vi "InsertOnMultipleWires.vi"(10 "Wire Array":refnum<vi>[](array[refnum]), 11 "To Insert":path) -> (2 "Inserted":refnum<vi>, 3 "Done?":bool)   [LabVIEW 2024, in "AddNewEvent.lvlib"]
uses:
  AddNewEvent.lvlib
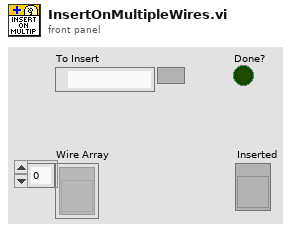
[diagram p1: front panel]
types:
  T1 = cluster{"Not Error Wire?":bool, "Source Term Top":i32, "Source Term Left":i32, "Wire Ref":refnum<vi>, "Source Term":refnum<vi>, "Sink Terms":refnum<vi>[], "Tried this one yet?":bool, "Sink Term Owner Owners":refnum<vi>[]}
  T2 = cluster{"Not Error Wire?":bool, "Source Term Top":i32, "Source Term Left":i32, "Wire Ref":refnum<vi>, "Source Term":refnum<vi>, "Sink Terms":refnum<vi>[], "Tried this one yet?":bool, "Sink Term Owner Owners":refnum<vi>[]}[]
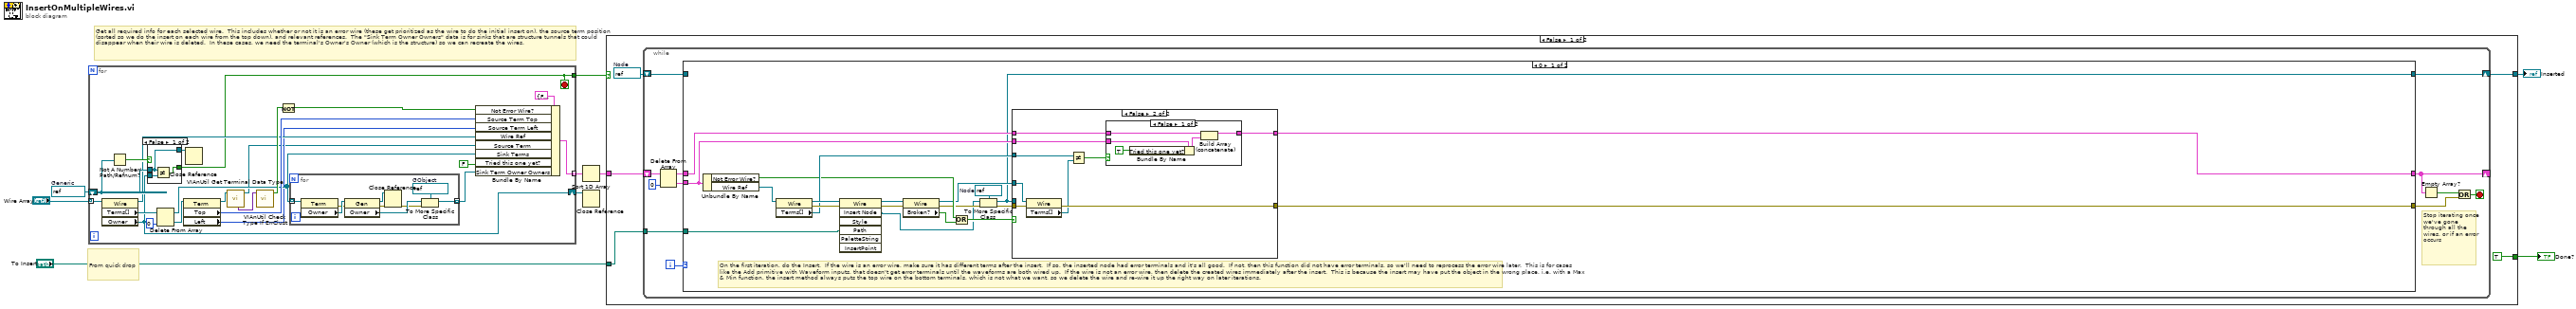
[diagram p0: block diagram]
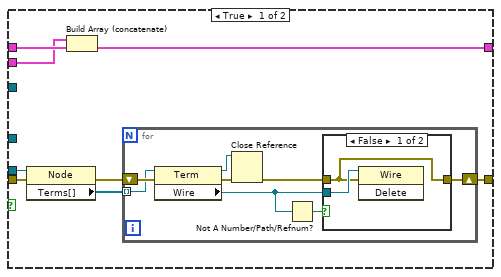
[diagram p2: hidden frame]
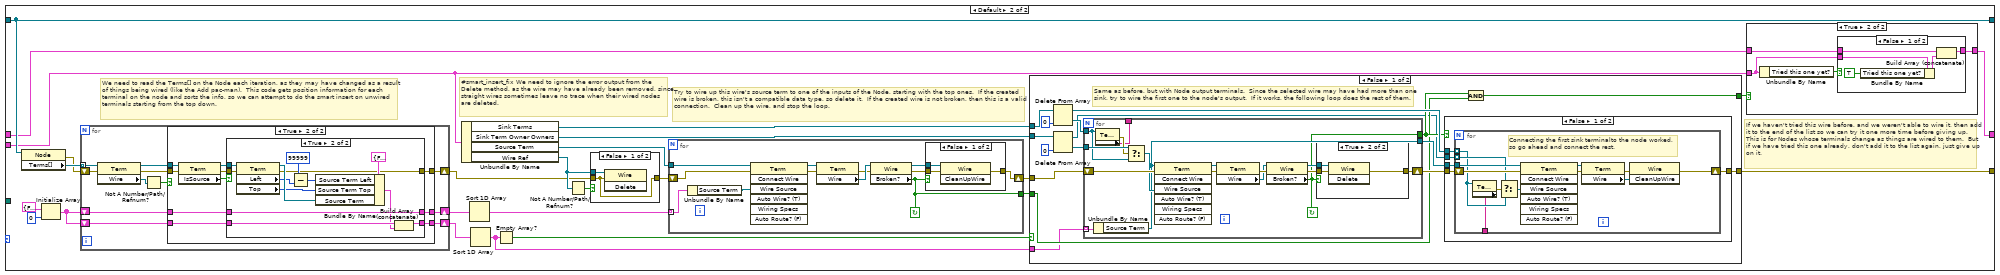
[diagram p5: hidden frame]
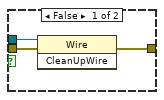
[diagram p8: hidden frame]
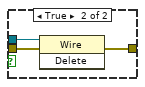
[diagram p12: hidden frame]
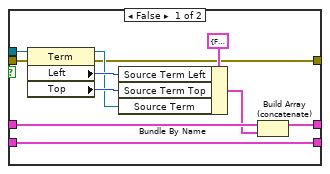
[diagram p14: hidden frame]
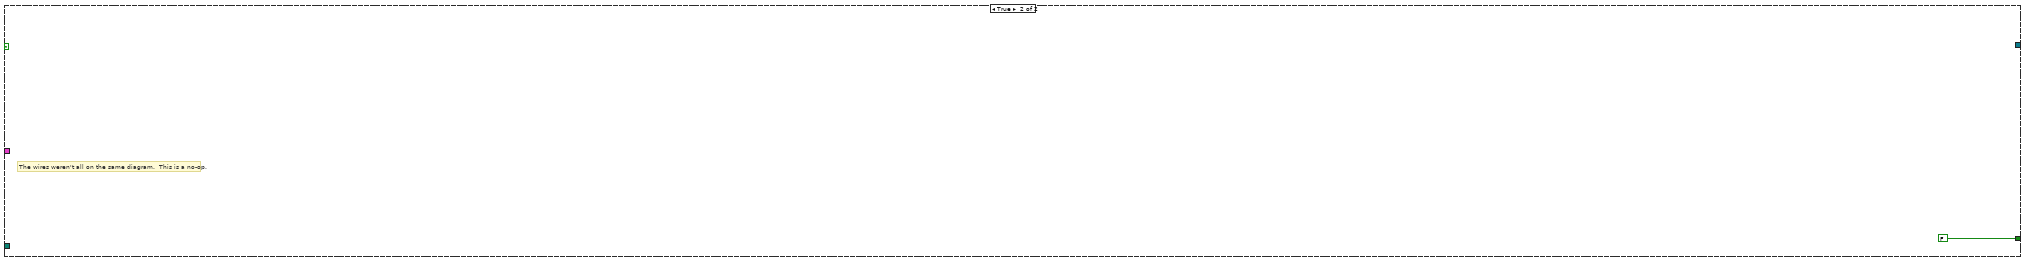
[diagram p15: hidden frame]
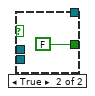
[diagram p16: hidden frame]
diagram:
  w6 = refnum<vi> refnum  # Generic
  # "From quick drop"
  # "Get all required info for each selected wire.  This includes whether or not it is an error wire (these get prioritized as the wire to do the initial insert on), the source term position (sorted so we do the insert on each wire from the top down), and relevant references.  The \"Sink Term Owner Owners\" data is for sinks that are structure tunnels that could disappear when their wire is deleted.  In these cases, we need the terminal's Owner's Owner (which is the structure) so we can recreate the wires."
  n1 = for {
    shift-right: [w16] -> w5
    shift-left: w6 -> [w31]
    tunnel: [w17] -> w7
    tunnel: "Wire Array" -> [w20] mode=indexing
    tunnel: [w19] -> w9 mode=indexing
    stop <- w17 stop-if-true
    n2 = property class="Wire"(reference=w20) -> (reference out=w23:refnum<vi>, "Terms[]"=w30:refnum<vi>[], "Owner"=w16:refnum<vi>)  [unwired: 1 in, 1 out]
    n3 = Not A Number/Path/Refnum?(number/path/refnum=w31) -> (NaN/Path/Refnum?=w28:bool)
    n4 = case shown="False" w28 {
      tunnel: [w42 FALSE] -> w17
      tunnel: w16 -> [w43 _]
      tunnel: w31 -> [w41 _]
      tunnel: [w41 _] -> w13
      frame False {
        n5 = Not Equal?(x=w41, y=w43) -> (x != y?=w42:bool)
      }
      frame True {
      }
    }
    n6 = Delete From Array(array=w30, index=0) -> (deleted portion=w18:refnum<vi>, array with subset deleted=w15:refnum<vi>[])  [unwired: 1 in]
    n7 = property class="Term"(reference=w18) -> (reference out=w12:refnum<vi>, "Top"=w25:i32, "Left"=w14:i32)  [unwired: 1 in, 1 out]
    n8 = Close Reference(reference=w13) -> ()  [unwired: 1 in, 1 out]
    n9 = call <vilib>:"VIAnUtil Get Terminal Data Type.vi"("Terminal in"=w12) -> ("Terminal out"=w11:refnum<vi>, "Type Variant"=w10:variant)  [unwired: 7 in, 2 out]
    n10 = call <vilib>:"VIAnUtil Check Type If ErrClust.vi"("Data In"=w10) -> ("IsErrClust?"=w26:bool)  [unwired: 1 in, 9 out]
    n11 = Not(x=w26) -> (.not. x?=w24:bool)
    n12 = for {
      tunnel: w15 -> [w40] mode=indexing
      tunnel: [w37] -> w21 mode=indexing
      w36 = refnum<vi> refnum  # GObject
      n13 = property class="Term"(reference=w40) -> (error out=w35:errorcluster, "Owner"=w39:refnum<vi>)  [unwired: 1 in, 1 out]
      n14 = property class="Gen"(reference=w39, error in=w35) -> (reference out=w33:refnum<vi>, error out=w34:errorcluster, "Owner"=w38:refnum<vi>)
      n15 = Close Reference(reference=w33, error in (no error)=w34) -> (error out=w32:errorcluster)
      n16 = To More Specific Class(target class=w36, reference=w38, error in=w32) -> (specific class reference=w37:refnum<vi>)  [unwired: 1 out]
    }
    n17 = Bundle By Name(cluster=T1 {"Not Error Wire?"=FALSE, "Source Term Top"=0, "Source Term Left"=0, "Wire Ref"=refnum, "Source Term"=refnum, "Sink Terms"=[], "Tried this one yet?"=FALSE, "Sink Term Owner Owners"=[]} ("Wire Information"), "Not Error Wire?"=w24, "Source Term Top"=w25, "Source Term Left"=w14, "Wire Ref"=w23, "Source Term"=w11, "Sink Terms"=w15, "Tried this one yet?"=FALSE, "Sink Term Owner Owners"=w21) -> (w19:T1)
  }
  n18 = Sort 1D Array(array=w9) -> (sorted array=w8:T2)
  n19 = Close Reference(reference=w5) -> ()  [unwired: 1 in, 1 out]
  n20 = case shown="False" w7 {
    tunnel: w8 -> [w49 _]
    tunnel: [TRUE FALSE] -> w2
    tunnel: "To Insert" -> [w46 _]
    tunnel: [w45 _] -> w1
    frame False {
      w48 = refnum<vi> refnum  # Node
      n21 = while {
        shift-right: [w59] -> _
        shift-left: w49 -> [w56]
        shift-right: [w51] -> w45
        shift-left: w48 -> [w58]
        tunnel: w46 -> [w52]
        i -> [w60]
        stop <- w53 stop-if-true
        # "Stop iterating once we've gone through all the wires, or if an error occurs"
        n22 = Delete From Array(array=w56, index=0) -> (deleted portion=w61:T1, array with subset deleted=w55:T2)  [unwired: 1 in]
        n23 = case shown="0" w60 {
          tunnel: w61 -> [w80 w125]
          tunnel: w55 -> [w68 w132]
          tunnel: [w62 w140] -> w51
          tunnel: [w81 w131] -> w59
          tunnel: w58 -> [_ w140]
          tunnel: [w79 w135] -> w50
          tunnel: w52 -> [w67 _]
          frame 0 {
            w65 = refnum<vi> refnum  # Node
            # "On the first iteration, do the Insert.  If the wire is an error wire, make sure it has different terms after the insert.  If so, the inserted node had error terminals and it's all good.  If not, then this function did not have error terminals, so we'll need to reprocess the error wire later.  This is for cases like the Add primitive with Waveform inputs, that doesn't get error terminals until the waveforms are both wired up.  If the wire is not an error wire, then delete the created wires immediately after the insert.  This is because the insert may have put the object in the wrong place, i.e. with a Max & Min function, the insert method always puts the top wire on the bottom terminals, which is not what we want, so we delete the wire and re-wire it up the right way on later iterations."
            n24 = Unbundle By Name(w80) -> ("Not Error Wire?"=w74:bool, "Wire Ref"=w78:refnum<vi>)
            n25 = property class="Wire"(reference=w78) -> (reference out=w76:refnum<vi>, error out=w77:errorcluster, "Terms[]"=w75:refnum<vi>[])  [unwired: 1 in]
            n26 = invoke class="Wire" method="Insert Node"(reference=w76, error in=w77, "Path"=w67) -> (reference out=w73:refnum<vi>, error out=w72:errorcluster, "Insert Node"=w63:refnum<vi>)  [unwired: 4 in, 4 out]
            n27 = property class="Wire"(reference=w73, error in=w72) -> (reference out=w71:refnum<vi>, error out=w66:errorcluster, "Broken?"=w70:bool)
            n28 = Or(x=w74, y=w70) -> (x .or. y?=w69:bool)
            n29 = To More Specific Class(target class=w65, reference=w63, error in=w66) -> (specific class reference=w62:refnum<vi>, error out=w64:errorcluster)
            n30 = case shown="False" w69 {
              tunnel: w68 -> [w89 w109]
              tunnel: [w87 w108] -> w81
              tunnel: w80 -> [w88 w107]
              tunnel: [w82 w104] -> w79
              tunnel: w64 -> [w84 w106]
              tunnel: w71 -> [_ w105]
              tunnel: w75 -> [_ w102]
              tunnel: w62 -> [w85 _]
              frame True {
                n31 = property class="Node"(reference=w85, error in=w84) -> (error out=w86:errorcluster, "Terms[]"=w83:refnum<vi>[])  [unwired: 1 out]
                n32 = Build Array (concatenate)(w88, w89) -> (w87:T2)
                n33 = for {
                  shift-right: [w91] -> w82
                  shift-left: w86 -> [w97]
                  tunnel: w83 -> [w96] mode=indexing
                  n34 = property class="Term"(reference=w96, error in=w97) -> (reference out=w94:refnum<vi>, error out=w95:errorcluster, "Wire"=w90:refnum<vi>)
                  n35 = Close Reference(reference=w94, error in (no error)=w95) -> (error out=w92:errorcluster)
                  n36 = Not A Number/Path/Refnum?(number/path/refnum=w90) -> (NaN/Path/Refnum?=w93:bool)
                  n37 = case shown="False" w93 {
                    tunnel: w92 -> [w98 w100]
                    tunnel: [w98 w100] -> w91
                    tunnel: w90 -> [w99 _]
                    frame False {
                      n38 = invoke class="Wire" method="Delete"(reference=w99, error in=w98) -> ()  [unwired: 1 in, 3 out]
                    }
                    frame True {
                    }
                  }
                }
              }
              frame False {
                n39 = property class="Wire"(reference=w105, error in=w106) -> (error out=w104:errorcluster, "Terms[]"=w103:refnum<vi>[])  [unwired: 1 out]
                n40 = Not Equal?(x=w102, y=w103) -> (x != y?=w101:bool)
                n41 = case shown="False" w101 {
                  tunnel: w109 -> [w114 w115]
                  tunnel: [w113 w115] -> w108
                  tunnel: w107 -> [w112 _]
                  frame False {
                    n42 = Bundle By Name(cluster=w112, "Tried this one yet?"=TRUE) -> (w111:T1)
                    n43 = Build Array (concatenate)(w114, w111) -> (w113:T2)
                  }
                  frame True {
                  }
                }
              }
            }
          }
          frame Default {
            # "#smart_insert_fix We need to ignore the error output from the Delete method, as the wire may have already been removed, since straight wires sometimes leave no trace when their wired nodes are deleted."
            # "If we haven't tried this wire before, and we weren't able to wire it, then add it to the end of the list so we can try it one more time before giving up.  This is for Nodes whose terminals change as things are wired to them.  But if we have tried this one already, don't add it to the list again, just give up on it."
            # "Try to wire up this wire's source term to one of the inputs of the Node, starting with the top ones.  If the created wire is broken, this isn't a compatible data type, so delete it.  If the created wire is not broken, then this is a valid connection.  Clean up the wire, and stop the loop."
            # "We need to read the Terms[] on the Node each iteration, as they may have changed as a result of things being wired (like the Add pac-man).  This code gets position information for each terminal on the node and sorts the info, so we can attempt to do the smart insert on unwired terminals starting from the top down."
            n44 = property class="Node"(reference=w140) -> (error out=w118:errorcluster, "Terms[]"=w139:refnum<vi>[])  [unwired: 1 in, 1 out]
            n45 = Initialize Array(T1 {"Not Error Wire?"=FALSE, "Source Term Top"=0, "Source Term Left"=0, "Wire Ref"=refnum, "Source Term"=refnum, "Sink Terms"=[], "Tried this one yet?"=FALSE, "Sink Term Owner Owners"=[]} ("Wire Information"), 0) -> (w119:T2)
            n46 = for {
              tunnel: w139 -> [w241] mode=indexing
              shift-right: [w237] -> w137
              shift-left: w119 -> [w240]
              shift-right: [w236] -> w136
              shift-left: w119 -> [w238]
              shift-right: [w231] -> w117
              shift-left: w118 -> [w233]
              n47 = property class="Term"(reference=w241, error in=w233) -> (reference out=w234:refnum<vi>, error out=w232:errorcluster, "Wire"=w235:refnum<vi>)
              n48 = Not A Number/Path/Refnum?(number/path/refnum=w235) -> (NaN/Path/Refnum?=w239:bool)
              n49 = case shown="True" w239 {
                tunnel: w240 -> [w244 w252]
                tunnel: w238 -> [w243 w251]
                tunnel: [w244 w249] -> w237
                tunnel: [w243 w250] -> w236
                tunnel: w234 -> [_ w254]
                tunnel: w232 -> [w242 w247]
                tunnel: [w242 w245] -> w231
                frame False {
                }
                frame True {
                  n50 = property class="Term"(reference=w254, error in=w247) -> (reference out=w248:refnum<vi>, error out=w246:errorcluster, "IsSource"=w253:bool)
                  n51 = case shown="True" w253 {
                    tunnel: w252 -> [w264 w276]
                    tunnel: w251 -> [w265 w278]
                    tunnel: [w265 w277] -> w250
                    tunnel: [w263 w276] -> w249
                    tunnel: w248 -> [w260 w275]
                    tunnel: w246 -> [w256 w268]
                    tunnel: [w255 w267] -> w245
                    frame False {
                      n52 = property class="Term"(reference=w260, error in=w256) -> (reference out=w257:refnum<vi>, error out=w255:errorcluster, "Left"=w259:i32, "Top"=w258:i32)
                      n53 = Bundle By Name(cluster=T1 {"Not Error Wire?"=FALSE, "Source Term Top"=0, "Source Term Left"=0, "Wire Ref"=refnum, "Source Term"=refnum, "Sink Terms"=[], "Tried this one yet?"=FALSE, "Sink Term Owner Owners"=[]} ("Wire Information"), "Source Term Left"=w259, "Source Term Top"=w258, "Source Term"=w257) -> (w261:T1)
                      n54 = Build Array (concatenate)(w264, w261) -> (w263:T2)
                    }
                    frame True {
                      n55 = property class="Term"(reference=w275, error in=w268) -> (reference out=w272:refnum<vi>, error out=w267:errorcluster, "Left"=w266:i32, "Top"=w271:i32)
                      n56 = Subtract(x=99999, y=w266) -> (x-y=w269:i32)
                      n57 = Bundle By Name(cluster=T1 {"Not Error Wire?"=FALSE, "Source Term Top"=0, "Source Term Left"=0, "Wire Ref"=refnum, "Source Term"=refnum, "Sink Terms"=[], "Tried this one yet?"=FALSE, "Sink Term Owner Owners"=[]} ("Wire Information"), "Source Term Left"=w269, "Source Term Top"=w271, "Source Term"=w272) -> (w273:T1)
                      n58 = Build Array (concatenate)(w278, w273) -> (w277:T2)
                    }
                  }
                }
              }
            }
            n59 = Unbundle By Name(w125) -> ("Sink Terms"=w124:refnum<vi>[], "Sink Term Owner Owners"=w123:refnum<vi>[], "Source Term"=w121:refnum<vi>, "Wire Ref"=w120:refnum<vi>)
            n60 = Sort 1D Array(array=w137) -> (sorted array=w130:T2)
            n61 = Sort 1D Array(array=w136) -> (sorted array=w129:T2)
            n62 = Empty Array?(array=w129) -> (empty?=w122:bool)
            n63 = Not A Number/Path/Refnum?(number/path/refnum=w120) -> (NaN/Path/Refnum?=w128:bool)
            n64 = case shown="False" w128 {
              tunnel: [w141 w143] -> w138
              tunnel: w120 -> [w142 _]
              tunnel: w117 -> [w141 w143]
              frame False {
                n65 = invoke class="Wire" method="Delete"(reference=w142, error in=w141) -> ()  [unwired: 1 in, 3 out]
              }
              frame True {
              }
            }
            n66 = for {
              tunnel: w121 -> [w224]
              tunnel: w130 -> [w223] mode=indexing
              tunnel: [w219] -> w133
              shift-right: [w213] -> w116
              shift-left: w138 -> [w217]
              stop <- w219 continue-if-true
              n67 = Unbundle By Name(w223) -> ("Source Term"=w218:refnum<vi>)
              n68 = invoke class="Term" method="Connect Wire"(reference=w224, error in=w217, "Wire Source"=w218) -> (reference out=w222:refnum<vi>, error out=w216:errorcluster)  [unwired: 4 in, 5 out]
              n69 = property class="Term"(reference=w222, error in=w216) -> (error out=w215:errorcluster, "Wire"=w221:refnum<vi>)  [unwired: 1 out]
              n70 = property class="Wire"(reference=w221, error in=w215) -> (reference out=w220:refnum<vi>, error out=w214:errorcluster, "Broken?"=w219:bool)
              n71 = case shown="False" w219 {
                tunnel: w220 -> [w227 w230]
                tunnel: w214 -> [w226 w229]
                tunnel: [w225 w228] -> w213
                frame False {
                  n72 = invoke class="Wire" method="CleanUpWire"(reference=w227, error in=w226) -> (error out=w225:errorcluster)  [unwired: 1 in, 2 out]
                }
                frame True {
                  n73 = invoke class="Wire" method="Delete"(reference=w230, error in=w229) -> (error out=w228:errorcluster)  [unwired: 1 in, 2 out]
                }
              }
            }
            n74 = case shown="False" w122 {
              tunnel: w124 -> [w159 _]
              tunnel: [w153 w200] -> w135
              tunnel: [w152 w201] -> w134
              tunnel: w133 -> [w150 w201]
              tunnel: w123 -> [w148 _]
              tunnel: w129 -> [w145 _]
              tunnel: w116 -> [w144 w200]
              frame False {
                # "Same as before, but with Node output terminals.  Since the selected wire may have had more than one sink, try to wire the first one to the node's output.  If it works, the following loop does the rest of them."
                n75 = Delete From Array(array=w159, index=0) -> (deleted portion=w157:refnum<vi>, array with subset deleted=w154:refnum<vi>[])  [unwired: 1 in]
                n76 = Delete From Array(array=w148, index=0) -> (deleted portion=w147:refnum<vi>, array with subset deleted=w146:refnum<vi>[])  [unwired: 1 in]
                n77 = for {
                  tunnel: w157 -> [w179]
                  tunnel: w145 -> [w184] mode=indexing
                  shift-right: [w186] -> w156
                  shift-left: w144 -> [w193]
                  tunnel: [w181] -> w151
                  tunnel: [w182] -> w155
                  tunnel: w147 -> [w185]
                  tunnel: [w178] -> _
                  stop <- w181 continue-if-true
                  n78 = Unbundle By Name(w184) -> ("Source Term"=w182:refnum<vi>)
                  n79 = property class="Term"(reference=w179) -> (error out=w180:errorcluster, "ClassName"=w178:string)  [unwired: 1 in, 1 out]
                  n80 = Select(t=w185, s=w180, f=w179) -> (s? t:f=w183:refnum<vi>)
                  n81 = invoke class="Term" method="Connect Wire"(reference=w182, error in=w193, "Wire Source"=w183) -> (reference out=w191:refnum<vi>, error out=w192:errorcluster)  [unwired: 4 in, 5 out]
                  n82 = property class="Term"(reference=w191, error in=w192) -> (error out=w190:errorcluster, "Wire"=w189:refnum<vi>)  [unwired: 1 out]
                  n83 = property class="Wire"(reference=w189, error in=w190) -> (reference out=w187:refnum<vi>, error out=w188:errorcluster, "Broken?"=w181:bool)
                  n84 = case shown="True" w181 {
                    tunnel: w188 -> [w196 w198]
                    tunnel: w187 -> [w195 w199]
                    tunnel: [w194 w197] -> w186
                    frame False {
                      n85 = invoke class="Wire" method="CleanUpWire"(reference=w195, error in=w196) -> (error out=w194:errorcluster)  [unwired: 1 in, 2 out]
                    }
                    frame True {
                      n86 = invoke class="Wire" method="Delete"(reference=w199, error in=w198) -> (error out=w197:errorcluster)  [unwired: 1 in, 2 out]
                    }
                  }
                }
                n87 = case shown="False" w151 {
                  tunnel: w156 -> [w164 w177]
                  tunnel: [w161 w177] -> w153
                  tunnel: w155 -> [w163 _]
                  tunnel: w154 -> [w162 _]
                  tunnel: w146 -> [w160 _]
                  frame False {
                    n88 = for {
                      tunnel: w163 -> [w175]
                      tunnel: w162 -> [w167] mode=indexing
                      shift-right: [w165] -> w161
                      shift-left: w164 -> [w176]
                      tunnel: w160 -> [w170] mode=indexing
                      tunnel: [w166] -> _
                      # "Connecting the first sink terminalto the node worked, so go ahead and connect the rest."
                      n89 = property class="Term"(reference=w167) -> (error out=w168:errorcluster, "ClassName"=w166:string)  [unwired: 1 in, 1 out]
                      n90 = Select(t=w170, s=w168, f=w167) -> (s? t:f=w169:refnum<vi>)
                      n91 = invoke class="Term" method="Connect Wire"(reference=w175, error in=w176, "Wire Source"=w169) -> (reference out=w174:refnum<vi>, error out=w173:errorcluster)  [unwired: 4 in, 5 out]
                      n92 = property class="Term"(reference=w174, error in=w173) -> (error out=w172:errorcluster, "Wire"=w171:refnum<vi>)  [unwired: 1 out]
                      n93 = invoke class="Wire" method="CleanUpWire"(reference=w171, error in=w172) -> (error out=w165:errorcluster)  [unwired: 1 in, 2 out]
                    }
                  }
                  frame True {
                    # "None of the node outputs would connect to this wire.  No need to try to process the rest of the sinks."
                  }
                }
                n94 = And(x=w151, y=w150) -> (x .and. y?=w152:bool)
              }
              frame True {
                # "There are no more unwired outputs on the node.  Don't bother trying to find one to wire to."
              }
            }
            n95 = case shown="True" w134 {
              tunnel: w132 -> [w202 w206]
              tunnel: w125 -> [_ w203]
              tunnel: [w202 w204] -> w131
              frame False {
              }
              frame True {
                n96 = Unbundle By Name(w203) -> ("Tried this one yet?"=w205:bool)
                n97 = case shown="False" w205 {
                  tunnel: w206 -> [w211 w212]
                  tunnel: [w210 w212] -> w204
                  tunnel: w203 -> [w209 _]
                  frame False {
                    n98 = Bundle By Name(cluster=w209, "Tried this one yet?"=TRUE) -> (w208:T1)
                    n99 = Build Array (concatenate)(w211, w208) -> (w210:T2)
                  }
                  frame True {
                  }
                }
              }
            }
          }
        }
        n100 = Empty Array?(array=w59) -> (empty?=w54:bool)
        n101 = Or(x=w54, y=w50) -> (x .or. y?=w53:bool)
      }
    }
    frame True {
      # "The wires weren't all on the same diagram.  This is a no-op."
    }
  }
  "Done?" <- w2
  "Inserted" <- w1
